vi "writeSaveData.vi"(8 "error in (no error)":errorcluster, 11 "reference in":refnum<class "excelFile.lvclass">) -> (0 "error out":errorcluster, 3 "reference out":refnum<class "excelFile.lvclass">)   [LabVIEW 2015, in "excelFile.lvclass"]
uses:
  excelFile.lvclass
  SYS/Devices Controller_llb/deviceType.ctl
  SYS/Items Controller_llb/storageSheets.ctl
  SYS/Devices Controller_llb/Devices Controller.lvclass
  SYS/Items Controller_llb/Items Controller.lvclass
panel:
  in  "storageSheets":T1
  in  "deviceType":T2
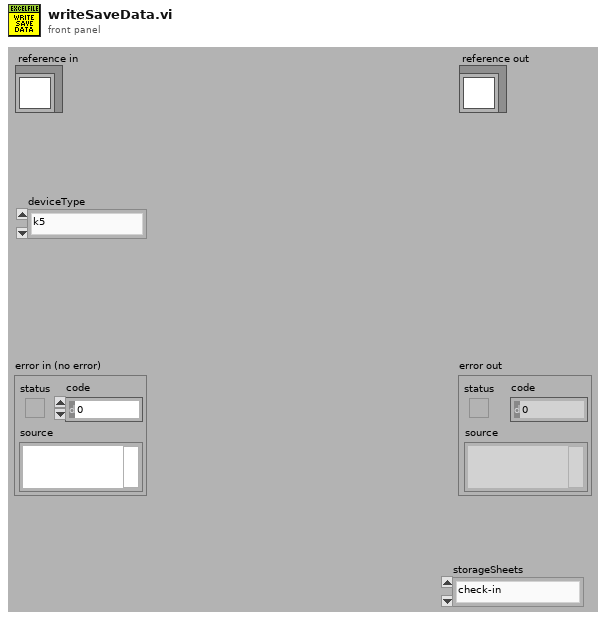
[diagram p1: front panel]
types:
  T1 = typedef "Items Controller.lvclass/storageSheets.ctl" = enum16{"check-in", "check-out", "storage"}
  T2 = typedef "Devices Controller.lvclass/deviceType.ctl" = enum16{"k5", "k4b2", "fitmate", "cpet", "rmr", "bodyBoxPft", "bp", "pp"}
  T3 = typedef "excelFile.lvclass/ObjectAttributesRef.ctl" = refnum<data-value>
  T4 = typedef "excelFile.lvclass/ObjectAttributes.ctl" = cluster{"MyAttribute":dbl, "path":string, "Refnum Excel":cluster{"Excel._Application":refnum<k7>, "Workbooks":refnum<k7>, "Open":refnum<k7>}, "data":string[][][], "save":bool, "fileType":T5, "rowsColor":u32[], "python_ref":refnum<class "python.lvclass">, "items_rows":i32[], "excel_range":i32[][], "TSR":cluster{"number":string, "TSR_path":path, "service_path":path, "email_to":string}}
  T5 = typedef "excelFile.lvclass/fileType.ctl" = enum16{"devices", "items", "partsTracking", "TSR"}
  T6 = cluster{"Excel._Application":refnum<k7>, "Workbooks":refnum<k7>, "Open":refnum<k7>}
  T7 = cluster{"Excel._Application":refnum<k7>, "Workbooks":refnum<k7>, "Open":refnum<k7>, "Worksheets":refnum<k7>, "Excel._Worksheet":refnum<k7>}
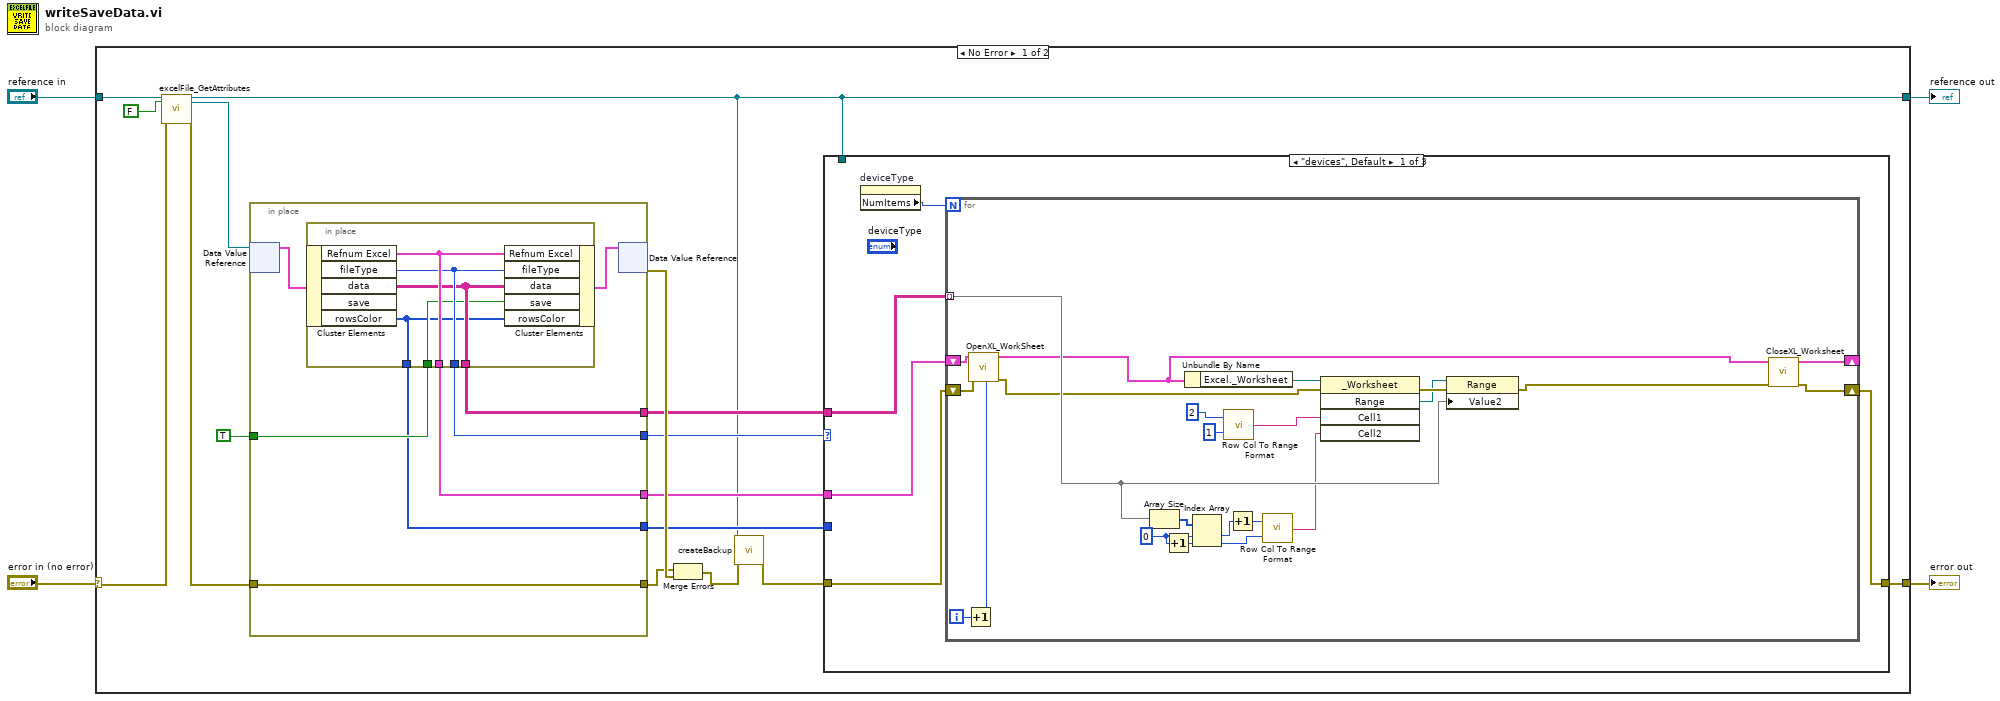
[diagram p0: block diagram]
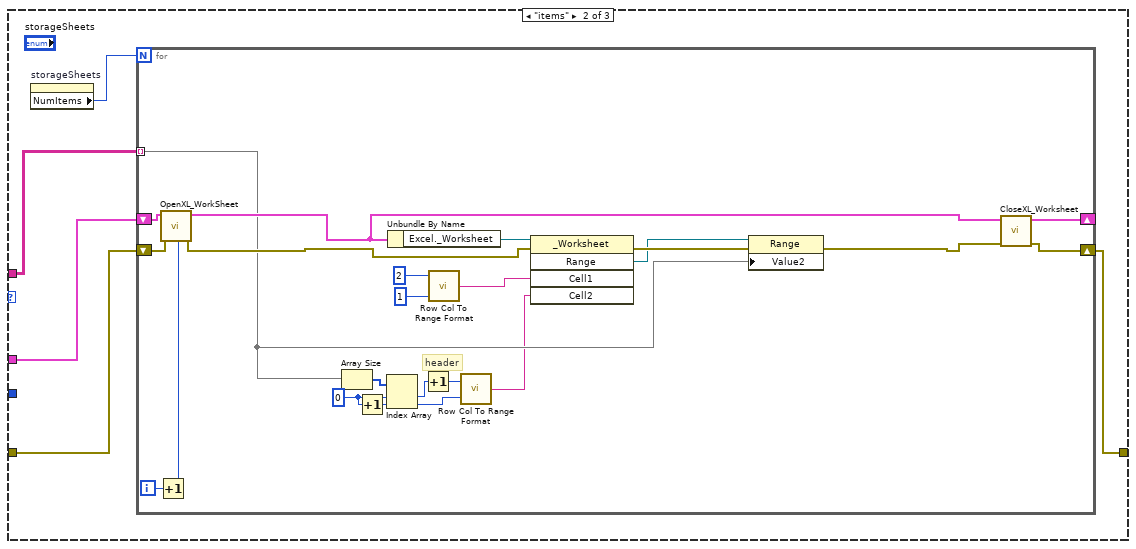
[diagram p2: hidden frame]
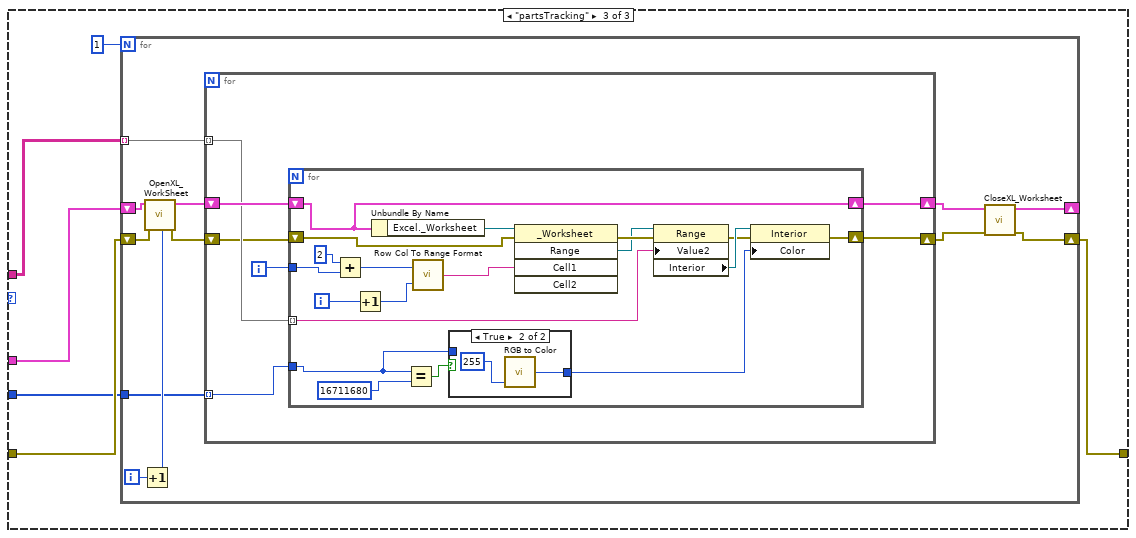
[diagram p3: hidden frame]
diagram:
  n1 = case shown="No Error" "error in (no error)" {
    selector: "error in (no error)" -> [w16 w138]
    tunnel: [w13 w138] -> w3
    tunnel: [w7 w137] -> w1
    tunnel: "reference in" -> [w18 w137]
    frame No Error {
      n2 = call "excelFile_GetAttributes.vi"("reference in"=w18, "return data? (T)"=FALSE, "error in (no error)"=w16) -> ("reference out"=w7:refnum<class "excelFile.lvclass">, "attributes ref"=w14:T3, "error out"=w15:errorcluster)  [unwired: 13 in, 1 out]
      n3 = in-place {
        in-place-border: w15 -> [w129]
        in-place-border: [w129] -> w19
        in-place-border: [w128] -> w12
        in-place-border: [w127] -> w11
        in-place-border: [w126] -> w10
        in-place-border: TRUE ("save") -> [w125]
        in-place-border: [w124] -> w8
        n4 = in-place-dvr #1(w14) -> (w130:T4)  [unwired: 1 out]
        n5 = in-place {
          in-place-border: [w136] -> w128
          in-place-border: [w135] -> w127
          in-place-border: [w134] -> w126
          in-place-border: w125 -> [w133]
          in-place-border: [w132] -> w124
          n6 = in-place-cluster #2(w130) -> ("Refnum Excel"=w136:T6, "fileType"=w135:T5, "data"=w134:string[][][], "rowsColor"=w132:u32[])  [unwired: 1 out]
          n7 = in-place-cluster #2("Refnum Excel"=w136, "fileType"=w135, "data"=w134, "save"=w133, "rowsColor"=w132) -> (w131:T4)
        }
        n8 = in-place-dvr #1(w131) -> (w20:errorcluster)  [unwired: 1 out]
      }
      n9 = Merge Errors(w19, w20) -> (w6:errorcluster)
      n10 = call "createBackup.vi"("reference in"=w7, "error in (no error)"=w6) -> ("error out"=w5:errorcluster)  [unwired: 16 in, 1 out]
      n11 = case shown="\"devices\", Default" w11 {
        tunnel: w5 -> [w22 w50 w80]
        tunnel: [w21 w49 w79] -> w13
        tunnel: w12 -> [w24 w51 w81]
        tunnel: w7 -> [_ _ _]
        tunnel: w10 -> [w23 w52 w82]
        tunnel: w8 -> [_ _ w77]
        frame "devices", Default {
          n12 = property on="deviceType" class="Enum (strict)"() -> ("NumItems"=w25:u32)  [unwired: 2 in, 2 out]
          n13 = for {
            N: w25 -> [_]
            tunnel: w23 -> [w48] mode=indexing
            shift-right: [w42] -> w21
            shift-left: w22 -> [w45]
            shift-right: [w41] -> _
            shift-left: w24 -> [w40]
            i -> [w46]
            w30 = 0 ("index")
            n14 = Increment(x=w46) -> (x+1=w39:i32)
            n15 = call <userlib>:"OpenXL_WorkSheet.vi"("Sheet"=w39, "error in (no error)"=w45, "Refnum Cluster In"=w40) -> ("error out"=w44:errorcluster, "Refnum Cluster Out"=w47:T7)  [unwired: 7 in]
            n16 = Array Size(array=w48) -> (size(s)=w33:i32[])
            n17 = Increment(x=w30) -> (x+1=w29:i32)
            n18 = Unbundle By Name(w47) -> ("Excel._Worksheet"=w38:refnum<k7>)
            n19 = Index Array(array=w33, index #1=w30, index #2=w29) -> (element #1=w32:i32, element #2=w31:i32)
            n20 = call <userlib>:"Row Col To Range Format.vi"("Column"=1, "Row"=2 ("x")) -> ("Output String"=w37:string)
            n21 = Increment(x=w32) -> (x+1=w26:i32)
            n22 = call <userlib>:"Row Col To Range Format.vi"("Column"=w31, "Row"=w26) -> ("Output String"=w28:string)
            n23 = invoke class="_Worksheet" method="Range"(reference=w38, error in=w44, "Cell1"=w37, "Cell2"=w28) -> (error out=w36:errorcluster, "Range"=w35:refnum<k7>)  [unwired: 1 in, 3 out]
            n24 = property class="Range"(reference=w35, error in=w36, "Value2"=w48) -> (error out=w43:errorcluster)  [unwired: 1 out]
            n25 = call <userlib>:"CloseXL_Worksheet.vi"("error in (no error)"=w43, "Refnum Cluster In"=w47) -> ("error out"=w42:errorcluster, "Refnum Cluster Out"=w41:T6)  [unwired: 8 in]
          }
        }
        frame "items" {
          n26 = property on="storageSheets" class="Enum (strict)"() -> ("NumItems"=w53:u32)  [unwired: 2 in, 2 out]
          n27 = for {
            N: w53 -> [_]
            tunnel: w52 -> [w56] mode=indexing
            shift-right: [w71] -> w49
            shift-left: w50 -> [w74]
            shift-right: [w70] -> _
            shift-left: w51 -> [w69]
            i -> [w75]
            w58 = 0 ("index")
            # "header"
            n28 = Increment(x=w75) -> (x+1=w68:i32)
            n29 = call <userlib>:"OpenXL_WorkSheet.vi"("Sheet"=w68, "error in (no error)"=w74, "Refnum Cluster In"=w69) -> ("error out"=w73:errorcluster, "Refnum Cluster Out"=w76:T7)  [unwired: 7 in]
            n30 = Array Size(array=w56) -> (size(s)=w61:i32[])
            n31 = Increment(x=w58) -> (x+1=w57:i32)
            n32 = Index Array(array=w61, index #1=w58, index #2=w57) -> (element #1=w60:i32, element #2=w59:i32)
            n33 = Unbundle By Name(w76) -> ("Excel._Worksheet"=w64:refnum<k7>)
            n34 = Increment(x=w60) -> (x+1=w54:i32)
            n35 = call <userlib>:"Row Col To Range Format.vi"("Column"=1 ("x"), "Row"=2 ("x")) -> ("Output String"=w67:string)
            n36 = call <userlib>:"Row Col To Range Format.vi"("Column"=w59, "Row"=w54) -> ("Output String"=w55:string)
            n37 = invoke class="_Worksheet" method="Range"(reference=w64, error in=w73, "Cell1"=w67, "Cell2"=w55) -> (error out=w66:errorcluster, "Range"=w65:refnum<k7>)  [unwired: 1 in, 3 out]
            n38 = property class="Range"(reference=w65, error in=w66, "Value2"=w56) -> (error out=w72:errorcluster)  [unwired: 1 out]
            n39 = call <userlib>:"CloseXL_Worksheet.vi"("error in (no error)"=w72, "Refnum Cluster In"=w76) -> ("error out"=w71:errorcluster, "Refnum Cluster Out"=w70:T6)  [unwired: 8 in]
          }
        }
        frame "partsTracking" {
          n40 = for {
            N: 1 -> [_]
            tunnel: w82 -> [w94] mode=indexing
            shift-right: [w87] -> w79
            shift-left: w80 -> [w91]
            shift-right: [w86] -> _
            shift-left: w81 -> [w85]
            tunnel: w77 -> [w83]
            i -> [w92]
            n41 = Increment(x=w92) -> (x+1=w84:i32)
            n42 = call <userlib>:"OpenXL_WorkSheet.vi"("Sheet"=w84, "error in (no error)"=w91, "Refnum Cluster In"=w85) -> ("error out"=w90:errorcluster, "Refnum Cluster Out"=w93:T7)  [unwired: 7 in]
            n43 = for {
              tunnel: w94 -> [w100] mode=indexing
              shift-right: [w98] -> w89
              shift-left: w93 -> [w101]
              shift-right: [w97] -> w88
              shift-left: w90 -> [w96]
              tunnel: w83 -> [w95] mode=indexing
              i -> [w99]
              n44 = for {
                tunnel: w100 -> [w117] mode=indexing
                tunnel: w99 -> [w115]
                shift-right: [w114] -> w98
                shift-left: w101 -> [w114]
                shift-right: [w106] -> w97
                shift-left: w96 -> [w113]
                tunnel: w95 -> [w102]
                i -> [w116]
                n45 = Add(x=2, y=w115) -> (x+y=w112:i32)
                n46 = Increment(x=w116) -> (x+1=w111:i32)
                n47 = Unbundle By Name(w114) -> ("Excel._Worksheet"=w109:refnum<k7>)
                n48 = Equal?(x=w102, y=u32 16711680) -> (x = y?=w104:bool)
                n49 = call <userlib>:"Row Col To Range Format.vi"("Column"=w111, "Row"=w112) -> ("Output String"=w120:string)
                n50 = case shown="True" w104 {
                  tunnel: [w121 w123] -> w103
                  tunnel: w102 -> [w121 _]
                  frame False {
                  }
                  frame True {
                    n51 = call <vilib>:"RGB to Color.vi"("B"=u8 255 ("R")) -> ("Color"=w123:u32)  [unwired: 2 in]
                  }
                }
                n52 = invoke class="_Worksheet" method="Range"(reference=w109, error in=w113, "Cell1"=w120) -> (error out=w119:errorcluster, "Range"=w118:refnum<k7>)  [unwired: 2 in, 3 out]
                n53 = property class="Range"(reference=w118, error in=w119, "Value2"=w117) -> (error out=w107:errorcluster, "Interior"=w108:refnum<k7>)  [unwired: 1 out]
                n54 = property class="Interior"(reference=w108, error in=w107, "Color"=w103) -> (error out=w106:errorcluster)  [unwired: 1 out]
              }
            }
            n55 = call <userlib>:"CloseXL_Worksheet.vi"("error in (no error)"=w88, "Refnum Cluster In"=w89) -> ("error out"=w87:errorcluster, "Refnum Cluster Out"=w86:T6)  [unwired: 8 in]
          }
        }
      }
    }
    frame Error {
    }
  }
  "error out" <- w3
  "reference out" <- w1
